vi "Open Shutter.vi"(8 "error in (no error)":errorcluster, 10 "Array":bool[](array[boolean]), 11 "Application in":refnum<class "Application.lvclass">) -> (0 "error out":errorcluster, 3 "Application out":refnum<class "Application.lvclass">)   [LabVIEW 2023, in "Application.lvlib" / "Application.lvclass"]
uses:
  Application.lvclass
  Application.lvclass/Application.ctl
  Hardware/Synchronization Device Messages/Set Shutter Enable Msg/Set Shutter Enable Msg.lvclass/Set Shutter Enable Msg.ctl
  <vilib>/ActorFramework/Message Enqueuer/Message Enqueuer.lvclass/Message Enqueuer.ctl
  User Interface/Main Window Messages/Shutter Status Update Msg/Shutter Status Update Msg.lvclass/Shutter Status Update Msg.ctl
  <vilib>/ActorFramework/Message Enqueuer/Enqueue.vi
  Hardware/Synchronization Device Messages/Set Shutter Enable Msg/Set Shutter Enable Msg.lvclass
  C:/Program Files/National Instruments/LabVIEW 2023/vi.lib/ActorFramework/Message/Message.lvclass
  User Interface/Main Window Messages/Shutter Status Update Msg/Shutter Status Update Msg.lvclass
  <vilib>/ActorFramework/Message Priority Queue/Priority Enqueue.vi
  Hardware/Sync Device/Sync Device/Synchronization Device Messages/Set Shutter Enable Msg/Set Shutter Enable Msg.lvclass
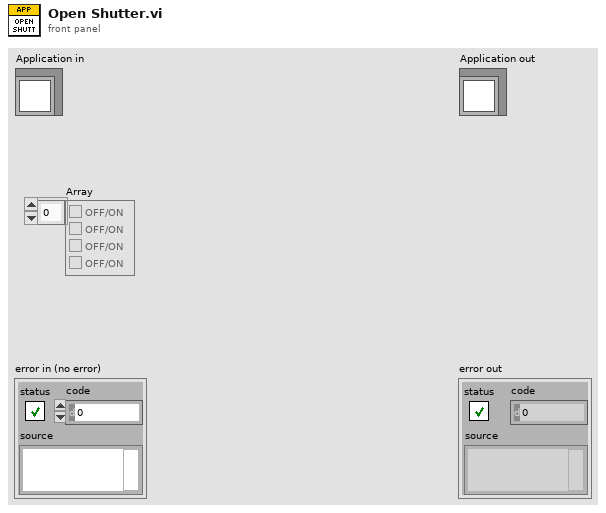
[diagram p1: front panel]
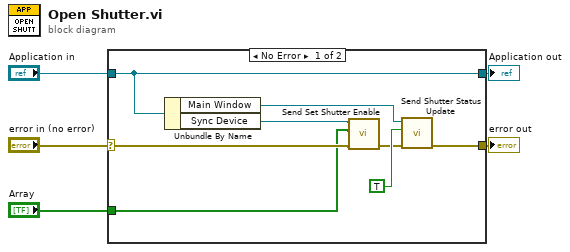
[diagram p0: block diagram]
diagram:
  n1 = case shown="No Error" "error in (no error)" {
    selector: "error in (no error)" -> [w7 w15]
    tunnel: [w12 w15] -> w4
    tunnel: [w13 w14] -> w2
    tunnel: "Application in" -> [w13 w14]
    tunnel: "Array" -> [w6 _]
    frame No Error {
      n2 = Unbundle By Name(w13) -> ("Main Window"=w10:refnum<class "Message Enqueuer.lvclass">, "Sync Device"=w8:refnum<class "Message Enqueuer.lvclass">)
      n3 = call "Send Set Shutter Enable.vi"("error in (no error)"=w7, "Shutter Enable"=w6, "Message Enqueuer"=w8) -> ("error out"=w9:errorcluster)  [unwired: 7 in, 1 out]
      n4 = call "Send Shutter Status Update.vi"("error in (no error)"=w9, "Shutters Active?"=TRUE, "Message Enqueuer"=w10) -> ("error out"=w12:errorcluster)  [unwired: 7 in, 1 out]
    }
    frame Error {
    }
  }
  "error out" <- w4
  "Application out" <- w2
